vi "Actor Core.vi"(8 "error in":errorcluster, 11 "IVI Oscilloscope in":refnum<class "IVI Oscilloscope.lvclass">) -> (0 "error out":errorcluster, 3 "Actor out":refnum<class "Actor.lvclass">)   [LabVIEW 2014, in "IVI Oscilloscope.lvclass"]
doc: "(<B>Filename</B>: Actor Framework.lvlib:Actor.lvclass:Actor Core.vi)\n\nReceives messages to the actor, reacts to them, and initiates any error handling that may shut the actor down.\n\nDescendant classes may override this VI to append parallel tasks for the actor to complete while it handles messages. Overrides use the Call Parent Method node."
uses:
  IVI Oscilloscope.lvclass
  Framework/Hardware/ReadoutDevice/ReadoutDevice.lvclass
  Framework/Interfaces/Observable Actor/Observable Actor.lvclass
  <vilib>/ActorFramework/Actor/Actor.lvclass
  Framework/Model/Data/Data1D/Data1D.lvclass
  Framework/Hardware/Device/Device Messages/Connect Msg/Connect Msg.lvclass
  Framework/Hardware/Device/Device Messages/Disconnect Msg/Disconnect Msg.lvclass
  Framework/Hardware/ReadoutDevice/ReadoutDevice Messages/Read Msg/Read Msg.lvclass
  Framework/Interfaces/Viewable Actor/Viewable Actor.lvclass
  IVI Oscilloscope Messages/Write Resource Name Msg/Write Resource Name Msg.lvclass
panel:
  in  "Disconnect":bool
  in  "Connect":bool
  in  "Read":bool
  out "Waveform Graph":waveform(dbl)(graph)
  in  "Resource Name":refnum<k15>
  out "Stop":bool=TRUE
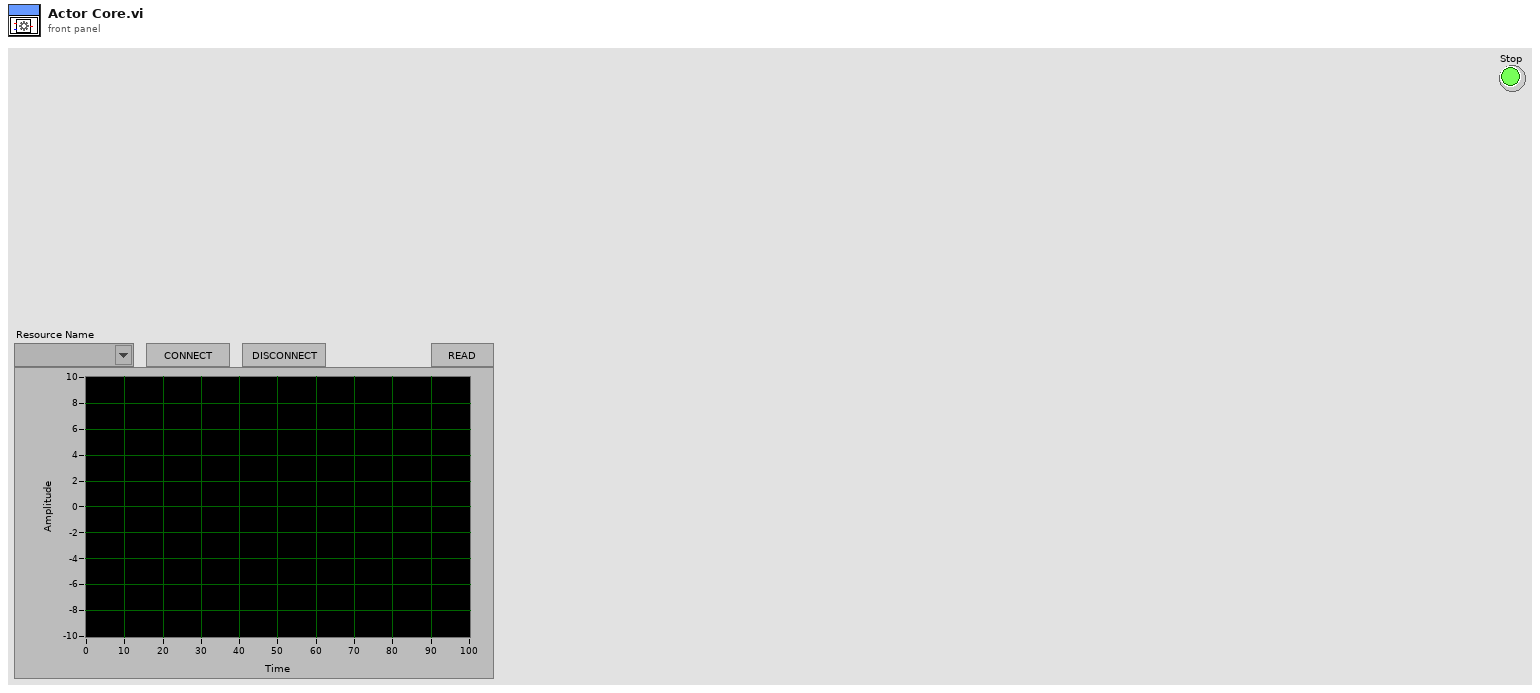
[diagram p1: front panel]
types:
  T1 = typedef "Observable Actor.lvlib/Observable Actor.lvclass/Observer.ctl" = refnum<queue>
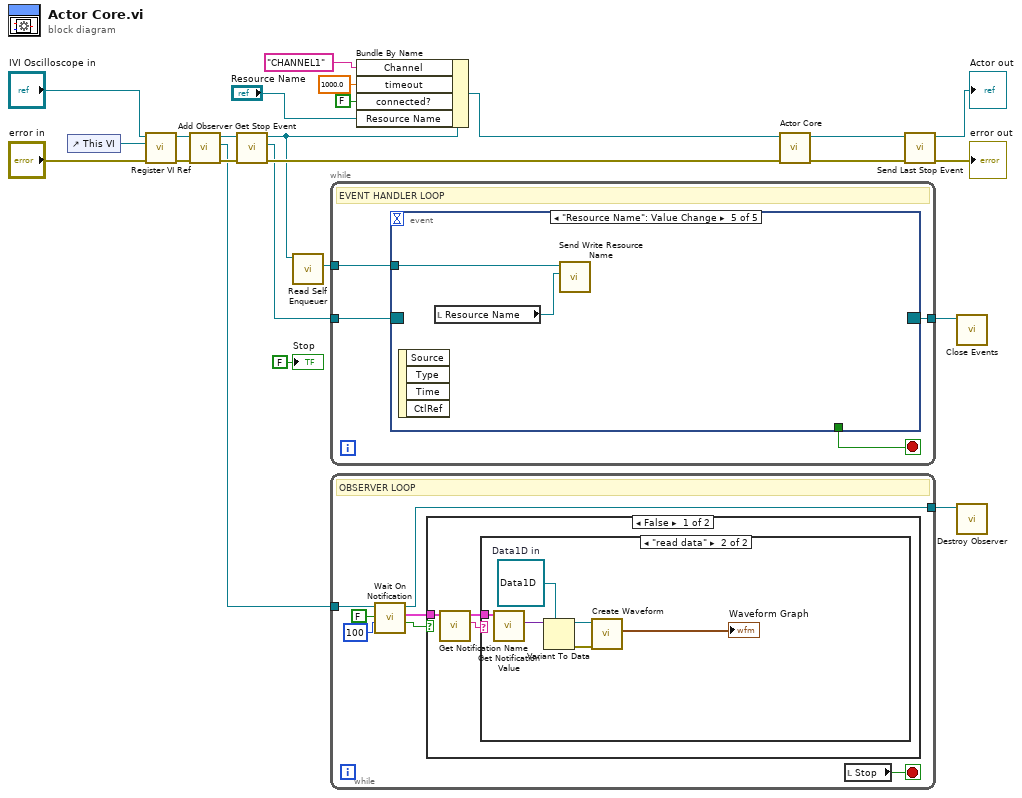
[diagram p0: block diagram]
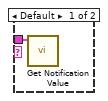
[diagram p2: hidden frame]
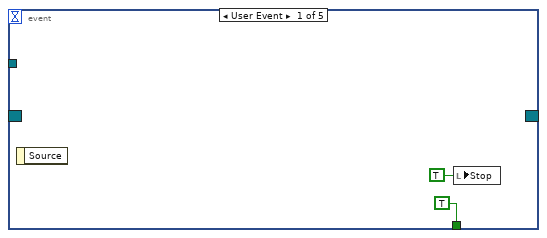
[diagram p4: hidden frame]
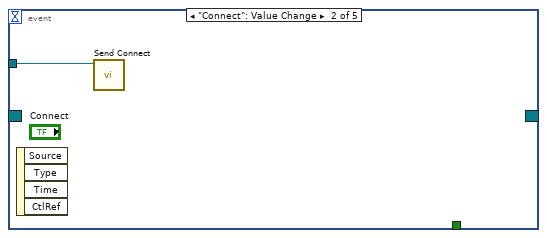
[diagram p5: hidden frame]
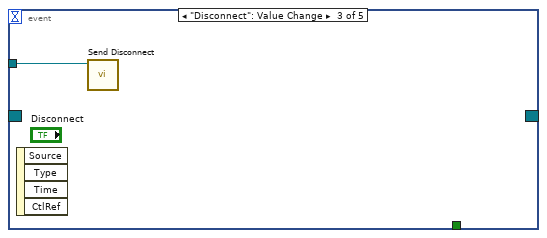
[diagram p6: hidden frame]
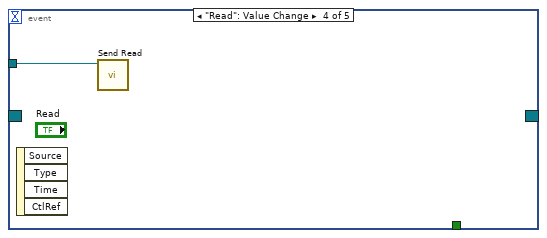
[diagram p7: hidden frame]
diagram:
  n1 = control-ref of="This VI"() -> (w1:refnum<vi>)
  n2 = call "Register VI Ref.vi"("error in (no error)"="error in", "VI ref"=w1, "Viewable Actor in"="IVI Oscilloscope in") -> ("error out"=w5:errorcluster, "Viewable Actor out"=w4:refnum<class "IVI Oscilloscope.lvclass">)  [unwired: 7 in]
  n3 = call-dynamic "Add Observer.vi"("error in (no error)"=w5, "Observable Actor in"=w4) -> ("error out"=w22:errorcluster, "new observer"=w14:T1, "Observable Actor out"=w23:refnum<class "IVI Oscilloscope.lvclass">)  [unwired: 7 in]
  n4 = call-dynamic "Get Stop Event.vi"("error in (no error)"=w22, "Observable Actor in"=w23) -> ("error out"=w19:errorcluster, "Events"=w16:refnum<event-registration>, "Observable Actor out"=w11:refnum<class "IVI Oscilloscope.lvclass">)  [unwired: 7 in]
  n5 = call <vilib>:"Read Self Enqueuer.vi"("Actor"=w11) -> ("Self Enqueuer"=w18:refnum<class "Message Enqueuer.lvclass">)  [unwired: 10 in]
  n6 = while {
    tunnel: w16 -> [w28]
    tunnel: w18 -> [w27]
    tunnel: [w26] -> w17
    stop <- w25 stop-if-true
    # "EVENT HANDLER LOOP"
    n7 = event shown="[4] \"Resource Name\": Value Change" {
      selector: w28 -> [_ _ _ _ _]
      dyn-events: [_ _ _ _ _] -> w26
      timeout: _ -> [_ _ _ _ _]
      tunnel: w27 -> [_ w31 w32 w33 w34]
      tunnel: [TRUE _ _ _ _] -> w25
      event User Event {
        n8 = event-data() -> ()  [unwired: 1 in, 1 out]
        n9 = local write "Stop"(TRUE ("Stop")) -> ()
      }
      event "Connect": Value Change {
        n10 = event-data() -> ()  [unwired: 1 in, 4 out]
        n11 = call "Send Connect.vi"("Message Enqueuer"=w31) -> ()  [unwired: 9 in, 2 out]
      }
      event "Disconnect": Value Change {
        n12 = event-data() -> ()  [unwired: 1 in, 4 out]
        n13 = call "Send Disconnect.vi"("Message Enqueuer"=w32) -> ()  [unwired: 9 in, 2 out]
      }
      event "Read": Value Change {
        n14 = event-data() -> ()  [unwired: 1 in, 4 out]
        n15 = call "Send Read.vi"("Message Enqueuer"=w33) -> ()  [unwired: 9 in, 2 out]
      }
      event "Resource Name": Value Change {
        n16 = event-data() -> ()  [unwired: 1 in, 4 out]
        n17 = local read "Resource Name"() -> (w35:refnum<k15>)
        n18 = call "Send Write Resource Name.vi"("Resource Name"=w35, "Message Enqueuer"=w34) -> ()  [unwired: 8 in, 2 out]
      }
    }
  }
  n19 = while {
    tunnel: w14 -> [w41]
    tunnel: [w38] -> w15
    stop <- w42 stop-if-true
    # "OBSERVER LOOP"
    n20 = call "Wait On Notification.vi"("timeout in ms (-1)"=100, "ignore previous (F)"=FALSE, "observer in"=w41) -> ("timed out?"=w36:bool, "notification"=w37:cluster{"value":variant, "name":string}, "observer out"=w38:T1)  [unwired: 5 in, 1 out]
    n21 = case shown="False" w36 {
      tunnel: w37 -> [w45 _]
      frame False {
        n22 = call "Get Notification Name.vi"("notification in"=w45) -> ("name"=w43:string, "notification out"=w44:cluster{"value":variant, "name":string})  [unwired: 9 in]
        n23 = case shown="\"read data\"" w43 {
          tunnel: w44 -> [w46 w52]
          frame Default {
            n24 = call "Get Notification Value.vi"("notification in"=w46) -> ()  [unwired: 7 in, 2 out]
          }
          frame "read data" {
            w50 = refnum<class "Data1D.lvclass"> refnum  # Data1D in
            n25 = call "Get Notification Value.vi"("notification in"=w52) -> ("data"=w51:variant)  [unwired: 7 in, 1 out]
            n26 = Variant To Data(type=w50, Variant=w51) -> (data=w49:refnum<class "Data1D.lvclass">, error out=w48:errorcluster)  [unwired: 1 in]
            n27 = call "Create Waveform.vi"("error in (no error)"=w48, "Data1D in"=w49) -> ("Waveform"=→"Waveform Graph":waveform(dbl))  [unwired: 7 in, 2 out]
          }
        }
      }
      frame True {
      }
    }
    n28 = local read "Stop"() -> (w42:bool)
  }
  n29 = Bundle By Name(cluster=w11, "Channel"="CHANNEL1" ("Settings.Channel"), "timeout"=1000.0, "connected?"=FALSE, "Resource Name"="Resource Name") -> (w9:refnum<class "IVI Oscilloscope.lvclass">)
  n30 = call-parent "Actor Core.vi"("error in"=w19, "Actor in"=w9) -> ("error out"=w20:errorcluster, "Actor out"=w21:refnum<class "Actor.lvclass">)  [unwired: 8 in]
  n31 = call "Send Last Stop Event.vi"("error in (no error)"=w20, "Actor in"=w21) -> ("error out"=→"error out":errorcluster, "Actor  out"=→"Actor out":refnum<class "Actor.lvclass">)  [unwired: 8 in]
  n32 = call "Close Events.vi"("events"=w17) -> ()  [unwired: 11 in]
  n33 = call "Destroy Observer.vi"("observer in"=w15) -> ()  [unwired: 11 in]
  "Stop" <- FALSE ("Stop")
